vi "connect to uut.vi"() -> ()   [LabVIEW 2015]
panel:
  out "standard output":string="['urllib.error.URLError =', ConnectionRefusedError(10061, 'No connection could be made because the target machine actively refused it', None, 10061, None)]\r\n"
  out "standard error":string
  out "return code":i32
  out "error out":errorcluster
  in  "command line":string="python urlx.py ConnectToScannerUnit(5)"
  in  "standard input":string
  in  "working directory":path=path "C:/Func Jobs/SnapOn/ModisEdge/Scanner/Test Sequence/TestScripts"
  in  "error in (no error)":errorcluster
  in  "wait until completion? (T)":bool=TRUE
  in  "run minimized? (F)":bool=TRUE
  in  "expected output size  (4096)":u32=4096
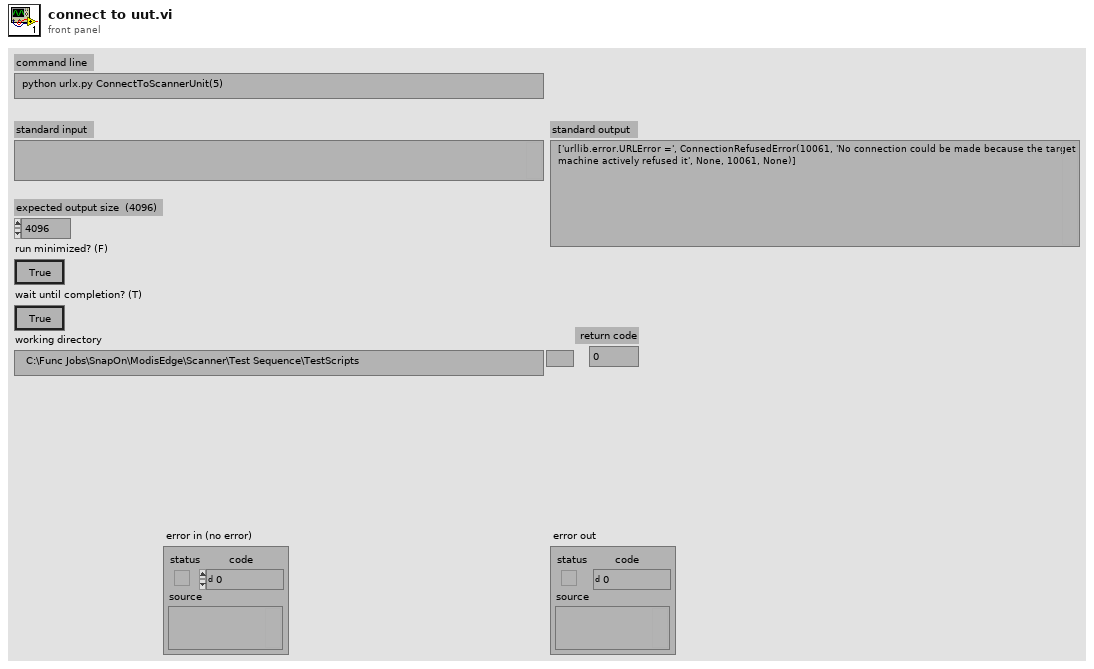
[diagram p1: front panel]
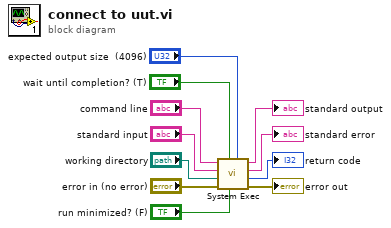
[diagram p0: block diagram]
diagram:
  n1 = call <vilib>:"System Exec.vi"("expected output size  (4096)"="expected output size  (4096)", "run minimized? (F)"="run minimized? (F)", "wait until completion? (T)"="wait until completion? (T)", "error in (no error)"="error in (no error)", "working directory"="working directory", "standard input"="standard input", "command line"="command line") -> ("error out"=→"error out":errorcluster, "return code"=→"return code":i32, "standard error"=→"standard error":string, "standard output"=→"standard output":string)  [unwired: 1 in]
